vi "test code emballage_ZEBRA_USB.vi"() -> ()   [LabVIEW 2011]
panel:
  in  "Nom de ressource VISA en sortie":refnum<visa-resource-name>="TLP2844Z"
  in  "chaine a ecrire":string="^XA\n~SD20\n^KL3\n^SC9600,8,N,1,,N\n^PRA\n^LL976\n^ML592\n^LH10,25\r\r^ADB,1,1^FT25,704^FDDestinataire : EMS Electro Medical System^FS\r^ADB,1,1^FT50,704^FDN§ commande : CF-08-0253/2^FS\r^ADB,1,1^FT75,704^FDQuantit‚ : 25/75^FS\r^ADB,1,1^FT100,704^FDVotre r‚f. : EL-360^FS\r^ADB,1,1^FT155,704^FDN§ valves :^FS\r^ADB,1,1^FT180,678^FD(P/N)^FS\r\r^FT390,40\n^BY1,2.0\n^BCI,56,N,N,N\n^FDEL-360 03 08010802 25^FS\r^AQI,1,1^FT390,10^FDEL-360 03 08010802 25^FS\r\r^A0B,18,18^FT155,568^FD 08010001,  08010002,  08010003,  08010004^FS\r^A0B,18,18^FT173,568^FD 08010005,  08010006,  08010007,  08010008^FS\r^A0B,18,18^FT191,568^FD 08010009,  08010010,  08010011,  08010012^FS\r^A0B,18,18^FT209,568^FD 08010013,  08010014,  08010015,  08010016^FS\r^A0B,18,18^FT227,568^FD 08010017,  08010018,  08010019,  08010020^FS\r^A0B,18,18^FT245,568^FD 08010022,  08010030,  08010099,  08020006^FS\r^A0B,18,18^FT263,568^FD 08020066^FS\r^A0B,18,18^FT281,568^FD ^FS\r^A0B,18,18^FT299,568^FD ^FS\r^A0B,18,18^FT317,568^FD ^FS\r\r^FT345,708\n^GB0,565,3^FS\n\n^FT501,708\n^BXB,4,0\n^FD12-216C-04521 EQIFIL 417mA 14.4ohm;03838/08-01.07.01;1/3^FS\r^ADB,1,1^FT388,568^FDN§ article FAS :^FS\r^AQB,1,1^FT418,568^FD12-216C-04521 EQIFIL 417mA 14.4ohm^FS\r^ADB,1,1^FT445,568^FDN§ commande FAS :^FS\r^AQB,1,1^FT475,568^FD03838/08-01.07.01^FS\r^ADB,1,1^FT500,568^FDCarton : ^FS\r^AQB,1,1^FT500,464^FD1/3^FS\r\r^PQ1\n^XZ\r"
  # "Grande etiquette - 1 code bar 2D + scan"
  # "Grande etiquette - 1 code bar 2D"
  # "ZB\nUS\nq592\nD7\nN\nR166,48\nI8,12,001\nA504,828,2,1,1,1,N,\"FASmedic s.a.\"\nA504,812,2,1,1,1,N,\"Zone industrielle\"\nA504,796,2,1,1,1,N,\"CH-1607 Pal‚zieux-Gare\"\nA504,780,2,1,1,1,N,\"T‚l.+41(0)21 907 79 71\"\nA504,764,2,1,1,1,N,\"www.fasmedic.com\"\nA34,712,3,2,1,1,N,\"Destinataire:EMS Electro Medical System\"\nA74,712,3,2,1,1,N,\"Nшcommande:CF-08-0253/2\"\nA114,712,3,2,1,1,N,\"Carton:1/2\"\nA154,712,3,2,1,1,N,\"Quantit‚:50/100\"\nA194,712,3,2,1,1,N,\"Votre ref.:EL-360\"\nLO258,112,2,600\nb404,112,D,4,\"12-216C-04521 EQIFIL 417mA 14.4ohm     03838/08-07.01.01\"\nA318,712,3,2,1,1,N,\"Nшarticle FAS:\"\nA358,712,3,3,1,1,N,\"12-216C-04521 EQIFIL 417mA 14.4ohm\"\nA398,712,3,2,1,1,N,\"Nшcommande FAS:\"\nA438,712,3,3,1,1,N,\"03838/08-07.01.01\"\nB318,64,2,3,1,2,56,N,\"EL-360 03 08010801\"\nA318,0,2,3,1,1,N,\"EL-360 03 08010801\"\nGW265,824,32,61,яяяяяяяяяяяяяяяяяяяяяяяяяяяяяяяЏяяяяяяяяяяяяяяяяяяяяяяяяяяяяяяюяяяяяяяяяяяяяяяяяяяяяяяяяяяяяяшяяяяяяяяяяяяяяяяяяяяяяяяяяяяяяАяяяяяяяяяяяяяяяяяяяяяяяяяяяяяяяяяяяяяяяяяяяяяяяяяяяяяяяяяяяяяяяяяяяяяяяяяяяяяяяяяяяяяяяяяюяяяяяяяяяяяяяяяяяяяяяяяяяяяяяюяяяяяяяяяяяяяяяяяяяяяяяяяяяяяюяяяяяяяяяяяяяяяяяяяяяяяяяяяяяьяяяяяяяяяяяяяяяяяяяяяяяяяяяяяьяяяяяяяяяяяяяяяяяяяяяяяяяяяяяшяЃяяяяьяяяяяяаяяяЂ?яяяяяяяшюП<ярьящяуя?Аяю8ш>П0x?БрьящяуьАяь0щяЏП#яЏь|ящяушАяшpуяЗП'яЏю<ящяурАяр`гягПяЏ?яящяуарАшяаазяуПяЗ?яњящяуашАьяЂАЗяуПяж?яњящяуашАьяАПяыПяжяЬящяуаяяАья~АяящПязяяМящяуаяяАшяЂяящП?язяяМящяуаяАаяЂяящП?ячяяМящяур?АяЂ?яящП?яцящяурАяА?яящП?яцящяушАяаяящП?яжяМящяуяАяряящПяжяЬящяуярАяяряяыПяжяњящягяяаАяяяшяПяуПяж?яњящягррАяяяяяяяяяяЗяуПяЗ?яясягррАшяяяяяяязягПяП?я>ясягрраряЂягязП'яЏџю>аяГраяЂ0ясяЏП#я‡ь~?А“шря0яшяП1ь?ГряЊ3ьшюpяь?П8аяЂsьью`яяЃяя?ѓяюяаяГяяАяяАяяьаяяяяя?яяяяяяяяяяяяяяяяяяьАяяяяя?яяяяяяяяяяяяяяяяяюьАяяяяя?яяяяяяяяяяяяяяяяяюшАяяяяя?яяяяяяяяяяяяяяяяяьшЂяяяяП?яяяяяяяяяяяяяяяяярЂяяяяП?яяяяяяяяяяяяяяяяяяр?яяяяП?яяяяяяяяяяяяяяяяяяр?яяяяП?яяяяяяяяяяяяяяяяяяаяяяяП?яяяяяяяяяяяяяяяяяяаяяяяяяяяяяяяяяяяяяяяяяяяАяяяяяяяяяяяяяяяяяяяяяяяяяяяАяяяяяяяяяяяяяяяяяяяяяяяяяяяЂяяяяяяяяяяяяяяяяяяяяяяяяяяяяяЂяяяяяяяяяяяяяяяяяяяяяяяяяяяяяЂ?яяяяяяяяяяяяяяяяяяяяяяяяяяяяяЂ?яяяяяяяяяяяяяяяяяяяяяяяяяяяяяЂ?яяяяяяяяяяяяяяяяяяяяяяяяяяяяяЂяяяяяяяяяяяяяяяяяяяяяяяяяяяяяАяяяяяяяяяяяяяяяяяяяяяяяяяяяяяаяяяяяяяяяяяяяяяяяяяяяяяяяяяяяяаяяяяяяяяяяяяяяяяяяяяяяяяяяяяяяряяяяяяяяяяяяяяяяяяяяяяяяяяяяяяр?яяяяяяяяяяяяяяяяяяяяяяяяяяяяяяшяяяяяяяяяяяяяяяяяяяяяяяяяяяяяящяяяяяя\nP1"
  # "FAS Medic RETOUR"
  # "FAS Medic normal"
  # "^XA\n^KL3\n^SC9600,8,N,1,,N\n^PRA\n^LL1428\n^ML888\n^MMC\n^LH300,90\n\n\n\n^AFB,1,1^FT0,940^FDDestinataire : EMS Electro Medical System^FS\n^AFB,1,1^FT40,940^FDN§ commande : CF-08-0253/2^FS\n^AFB,1,1^FT80,940^FDQuantit‚ : 25/25^FS\n^AFB,1,1^FT120,940^FDVotre r‚f. : EL-360^FS\n^AFB,1,1^FT200,940^FDN§ valves :^FS\n^AFB,1,1^FT235,905^FD(P/N)^FS\n\n^FT630,30\n^BY2,2.0\n^BCI,80,N,N,N\n^FD MK01852  09 08010802 50^FS\n^A0I,30,30^FT485,0^FD MK01852  09 08010802 50^FS\n\n^A0B,24,24^FT200,750^FD 08010001,  08010002,  08010003,  08010004,  08010004^FS\n^A0B,24,24^FT225,750^FD 08010005,  08010006,  08010007,  08010008,  08010004^FS\n^A0B,24,24^FT250,750^FD 08010009,  08010010,  08010011,  08010012,  08010004^FS\n^A0B,24,24^FT275,750^FD 08010013,  08010014,  08010015,  08010016,  08010004^FS\n^A0B,24,24^FT300,750^FD 08010017,  08010018,  08010019,  08010020,  08010004^FS\n^A0B,24,24^FT325,750^FD 08010022,  08010030,  08010099,  08020006,  08010004^FS\n^A0B,24,24^FT350,750^FD 08010022,  08010030,  08010099,  08020006,  08010004^FS\n^A0B,24,24^FT375,750^FD 08010022,  08010030,  08010099,  08020006,  08010004^FS\n^A0B,24,24^FT400,750^FD 08010022,  08010030,  08010099,  08020006,  08010004^FS\n^A0B,24,24^FT425,750^FD 08010022,  08010030,  08010099,  08020006,  08010004^FS\n\n^FT465,940\n^GB0,800,3^FS\n\n^FT650,940\n^BXB,6,0\n^FD12-216C-04521 EQIFIL 417mA 14.4ohm;03838/08-01.07.01;1/1^FS\n^AFB,1,1^FT525,760^FDN§ article FAS :^FS\n^A0B,30,30^FT560,760^FD12-216C-04521 EQIFIL 417mA 14.4ohm^FS\n^AFB,1,1^FT595,760^FDN§ commande FAS :^FS\n^A0B,30,30^FT630,760^FD03838/08-01.07.01^FS\n^AFB,1,1^FT665,760^FDCarton : ^FS\n^A0B,30,30^FT665,616^FD1/1^FS\n\n^PQ1\n^XZ"
  # "^XA\n^KL3\n^SC9600,8,N,1,,N\n^PRA\n^LL1428\n^ML888\n^MMC\n^LH300,90\n\n\n\n^AFB,1,1^FT0,940^FDDestinataire : EMS Electro Medical System^FS\n^AFB,1,1^FT40,940^FDN§ commande : CF-08-0253/2^FS\n^AFB,1,1^FT80,940^FDQuantit‚ : 25/25^FS\n^AFB,1,1^FT120,940^FDVotre r‚f. : EL-360^FS\n^AFB,1,1^FT200,940^FDN§ valves :^FS\n^AFB,1,1^FT235,905^FD(P/N)^FS\n\n^AVI,1,1^FT370,26^FDRETOUR^FS\n\n^A0B,24,24^FT200,750^FD 08010001,  08010002,  08010003,  08010004^FS\n^A0B,24,24^FT225,750^FD 08010005,  08010006,  08010007,  08010008^FS\n^A0B,24,24^FT250,750^FD 08010009,  08010010,  08010011,  08010012^FS\n^A0B,24,24^FT275,750^FD 08010013,  08010014,  08010015,  08010016^FS\n^A0B,24,24^FT300,750^FD 08010017,  08010018,  08010019,  08010020^FS\n^A0B,24,24^FT325,750^FD 08010022,  08010030,  08010099,  08020006^FS\n^A0B,24,24^FT350,750^FD 08010022^FS\n^A0B,24,24^FT375,750^FD^FS\n^A0B,24,24^FT400,750^FD^FS\n^A0B,24,24^FT425,750^FD^FS\n\n^FT465,940\n^GB0,800,3^FS\n\n^FT650,940\n^BXB,6,0\n^FD12-216C-04521 EQIFIL 417mA 14.4ohm;R03838/08-01.07.01;1/1^FS\n^AFB,1,1^FT525,760^FDN§ article FAS :^FS\n^A0B,30,30^FT560,760^FD12-216C-04521 EQIFIL 417mA 14.4ohm^FS\n^AFB,1,1^FT595,760^FDN§ commande FAS :^FS\n^A0B,30,30^FT630,760^FDR03838/08-01.07.01^FS\n^AFB,1,1^FT665,760^FDCarton : ^FS\n^A0B,30,30^FT665,616^FD1/1^FS\n\n^PQ1\n^XZ"
  # "^XA\n^KL3\n^SC9600,8,N,1,,N\n^PRA\n^LH0,0\n^LL960\n^ML592\n^FO50,50\n^ADN,36,20\n^FDDestinataire^FS\n^PQ1\n^XZ"
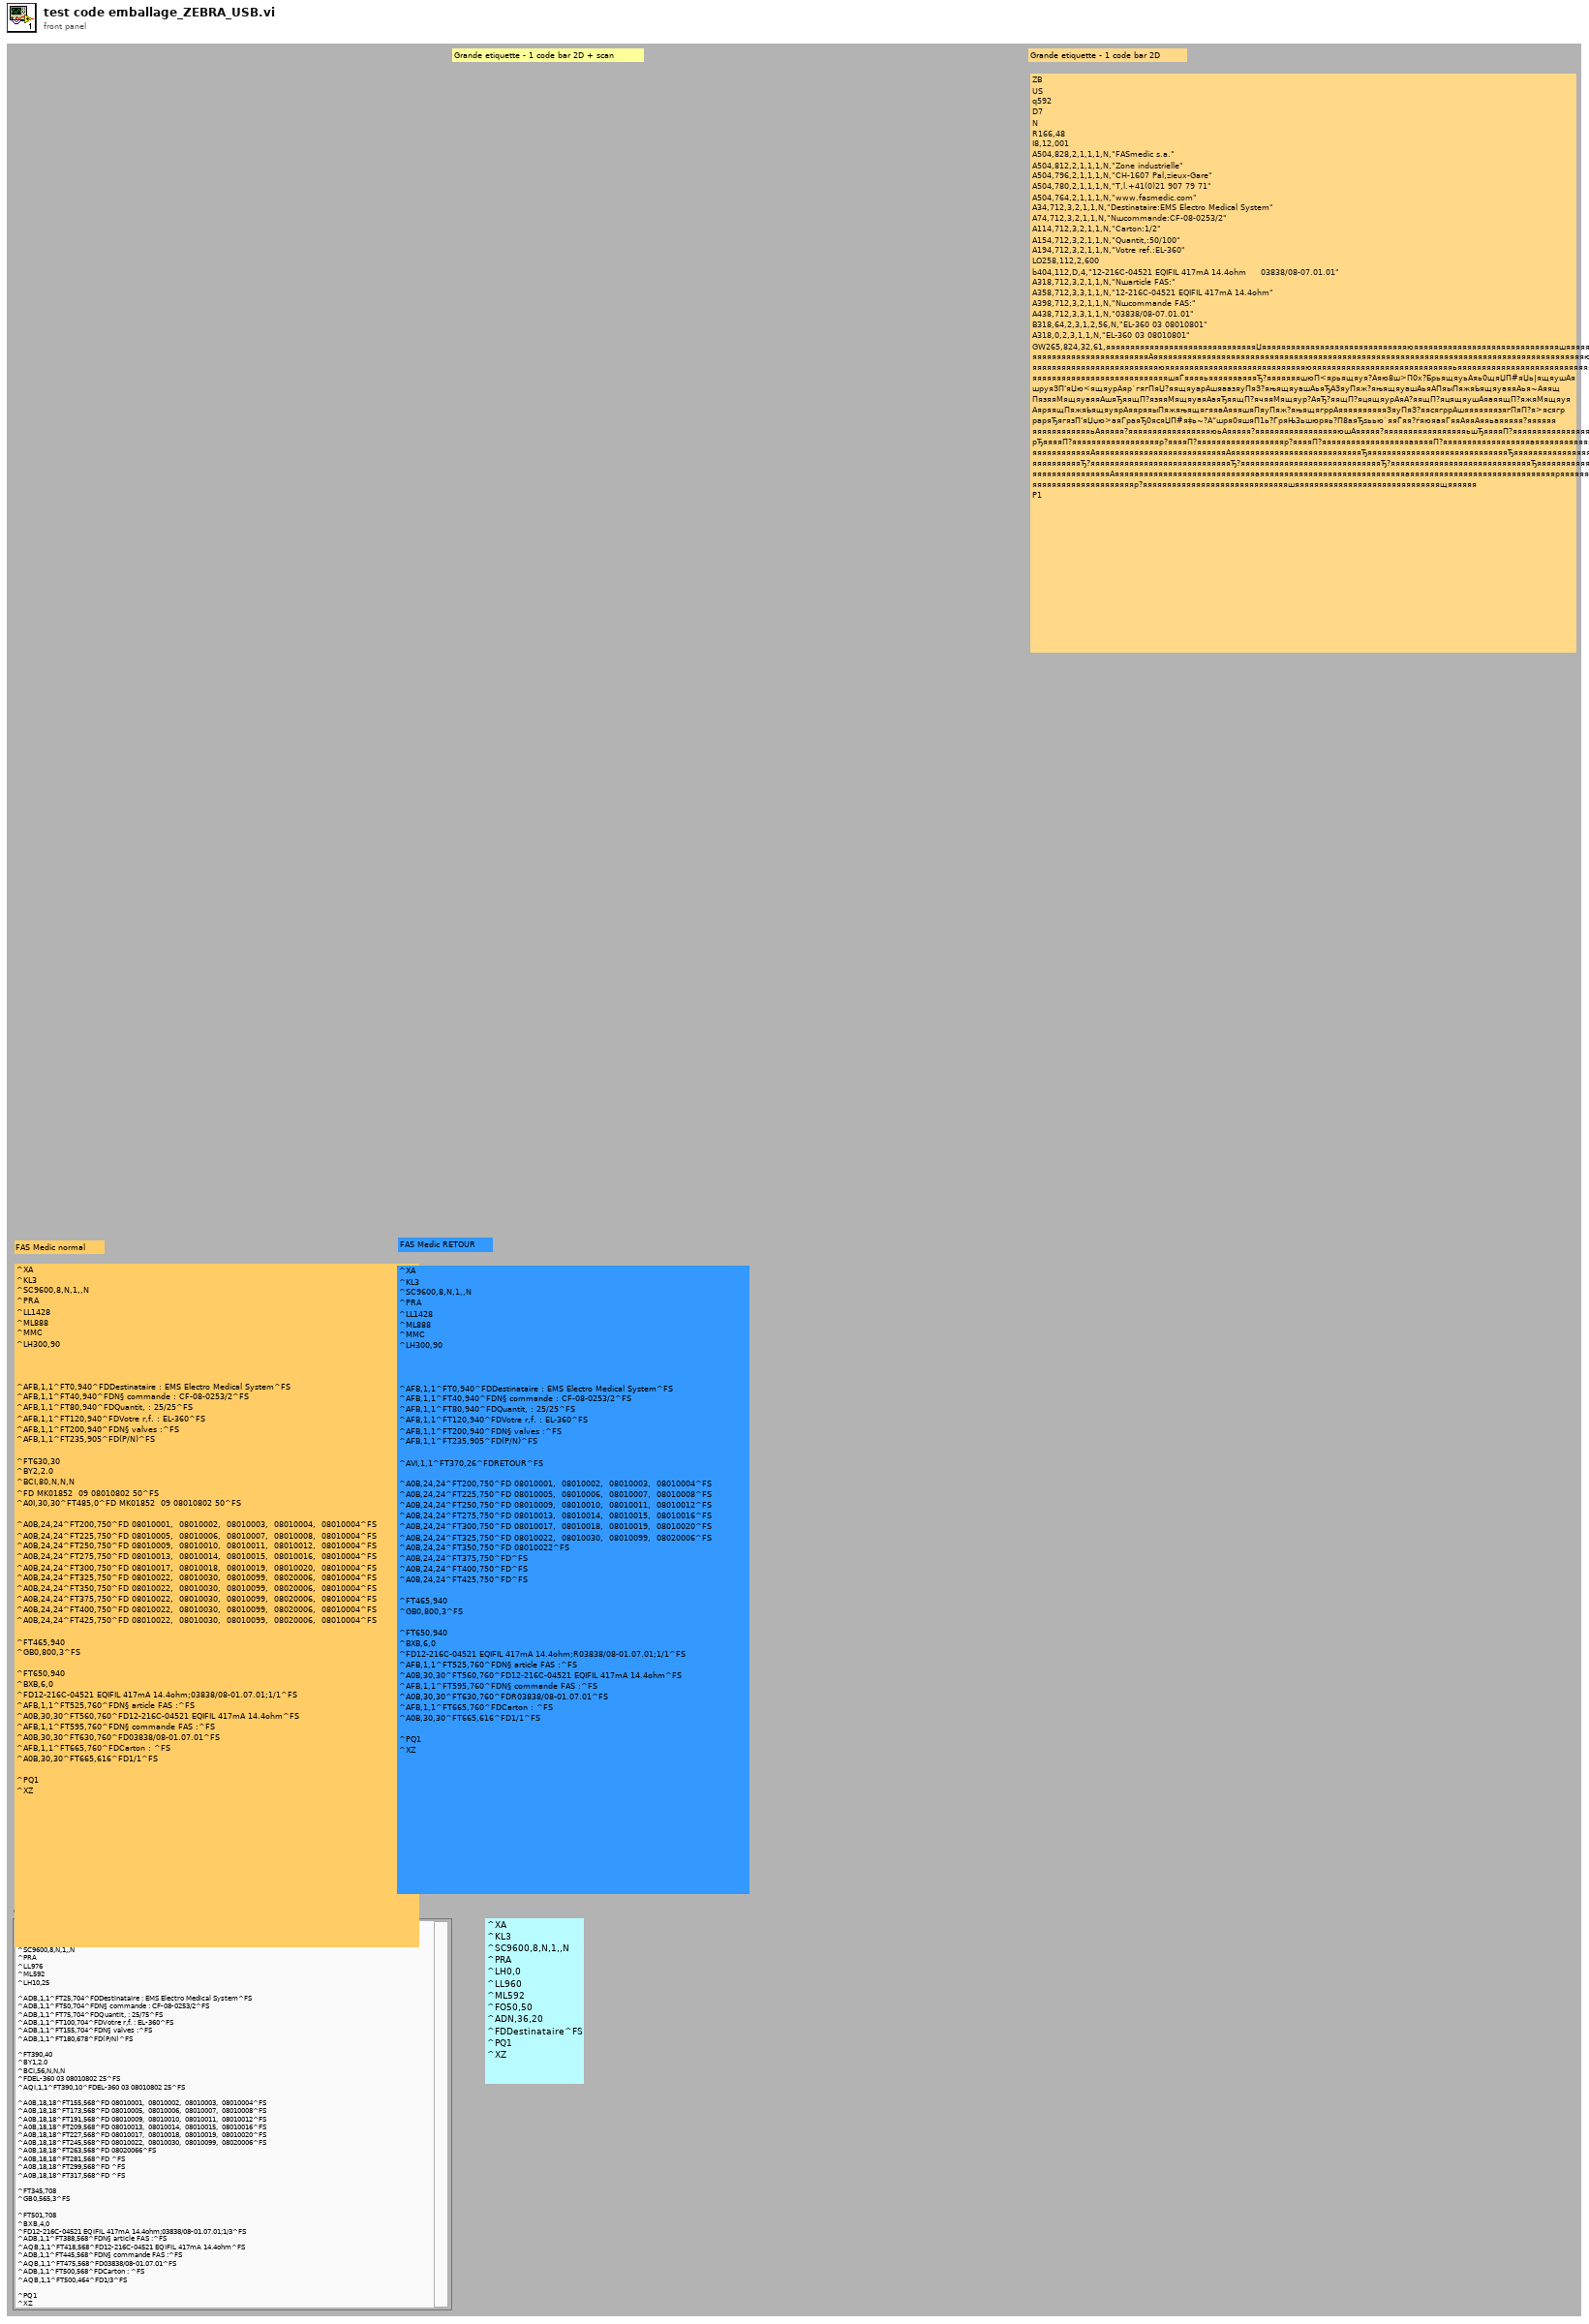
[diagram p1: front panel]
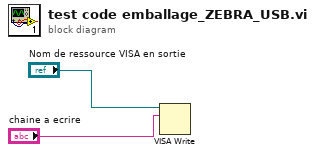
[diagram p0: block diagram]
diagram:
  n1 = VISA Write(VISA resource name="Nom de ressource VISA en sortie", write buffer="chaine a ecrire") -> ()  [unwired: 1 in, 3 out]
